vi "Accept_Only_Lvfiles.vi"(8 "error in (no error)":errorcluster, 11 "AB_Destination in":refnum<class "AB_Destination.lvclass">) -> (0 "error out":errorcluster, 2 "onlyLVfiles":bool, 3 "AB_Destination out":refnum<class "AB_Destination.lvclass">)   [LabVIEW 2020, in "AB_Destination.lvclass"]
uses:
  <vilib>/AppBuilder/AB_Classes/Destination/AB_Destination.lvclass
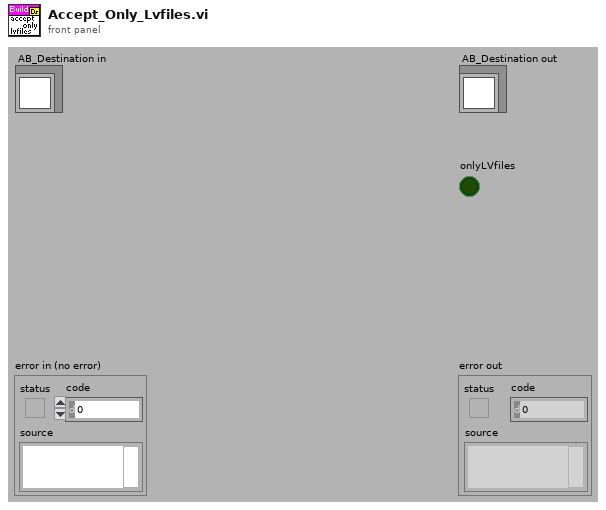
[diagram p1: front panel]
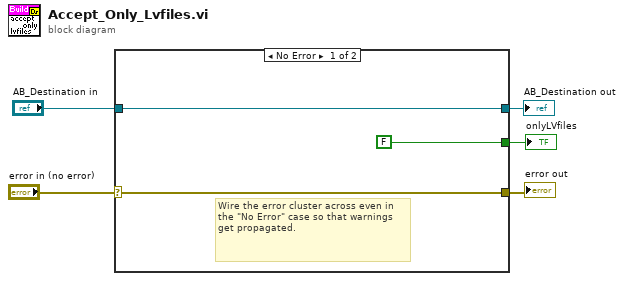
[diagram p0: block diagram]
diagram:
  n1 = case shown="No Error" "error in (no error)" {
    selector: "error in (no error)" -> [w7 w10]
    tunnel: [w7 w10] -> w4
    tunnel: [w8 w9] -> w2
    tunnel: "AB_Destination in" -> [w8 w9]
    tunnel: [FALSE _] -> w1
    frame No Error {
      # "Wire the error cluster across even in the \"No Error\" case so that warnings get propagated."
    }
    frame Error {
    }
  }
  "error out" <- w4
  "AB_Destination out" <- w2
  "onlyLVfiles" <- w1
